vi "test_outfrq_fpga_1x_clc.vi"() -> ()   [LabVIEW 2013]
uses:
  <vilib>/Platform/TimedLoop/XDataNode/timing_clust.ctl
  <vilib>/Platform/TimedLoop/XDataNode/nitl_modes.ctl
  <vilib>/Platform/TimedLoop/XDataNode/wakeup.ctl
  <vilib>/rvi/Emulation/niFpgaSctlEmulationGetInTimedLoop.vi
  <vilib>/rvi/Emulation/niFpgaEmulationReportErrorSimple.vi
  <vilib>/rvi/Emulation/niFpgaGetClockAttributes.vi
  <vilib>/rvi/eio/common/nirviEmuTemplateMethod_errors.vi
  <vilib>/rvi/Emulation/niFpgaCriticalErrorInLSC.vi
  <vilib>/Platform/TimedLoop/XDataNode/XDataNode.xnode
  <vilib>/eio/EIONode/EIONode.xnode
  <vilib>/Platform/TimedLoop/XDataNode/XDNodeRunTimeDep.lvlib
panel:
  out "IO Module\\User Error":u8
  in  "use AO1":bool
  in  "User Command Commit":bool
  in  "User Command":u8
  out "User Command Idle":bool
  out "User Command Status":u8
  in  "User Data 0":u8
  in  "User Data 1":u8
  out "PLL Locked":bool
  out "Configured?":bool
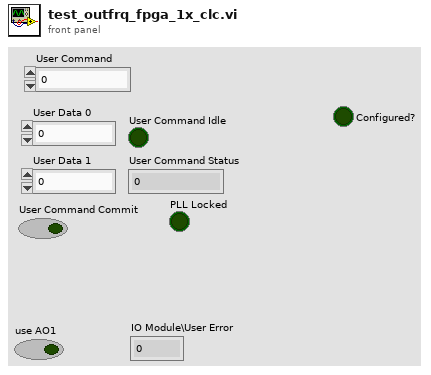
[diagram p1: front panel]
types:
  T1 = typedef "XDNodeRunTimeDep.lvlib/timing_clust.ctl" = cluster{"Expected End [f-1]":u64, "Actual End [f-1]":u64, "Finished Late? [f-1]":bool, "Expected End [i-1]":u64, "Actual End [i-1]":u64, "Finished Late? [i-1]":bool, "Expected Start [i]":u64, "Actual Start [i]":u64, "Expected Start [f]":u64, "Actual Start [f]":u64, "Source Name":string, "Structure Name":string, "Period":i64, "Deadline":i64, "Offset":i64, "Start":i64, "Priority":i32, "Timeout":i32, "Mode":T2, "Wakeup Reason":T3, "Error":errorcluster, "Source Type":string, "Secondary Source Type":string, "Global End Time":u64, "Global Start Time":u64, "Frame Duration":u64, "Iteration Duration":u64, "Assigned CPU":i32, "I/O Scan Engine Mode":u32}
  T2 = typedef "XDNodeRunTimeDep.lvlib/nitl_modes.ctl" = enum32{"No Change", "Process missed periods, maintain original phase", "Discard missed periods, maintain original phase", "Process missed periods, ignore original phase", "Discard missed periods, ignore original phase"}
  T3 = typedef "XDNodeRunTimeDep.lvlib/wakeup.ctl" = enum32{"Normal", "Aborted", "Asynchronous wakeup", "Timing source error", "Timed loop error", "Timeout"}
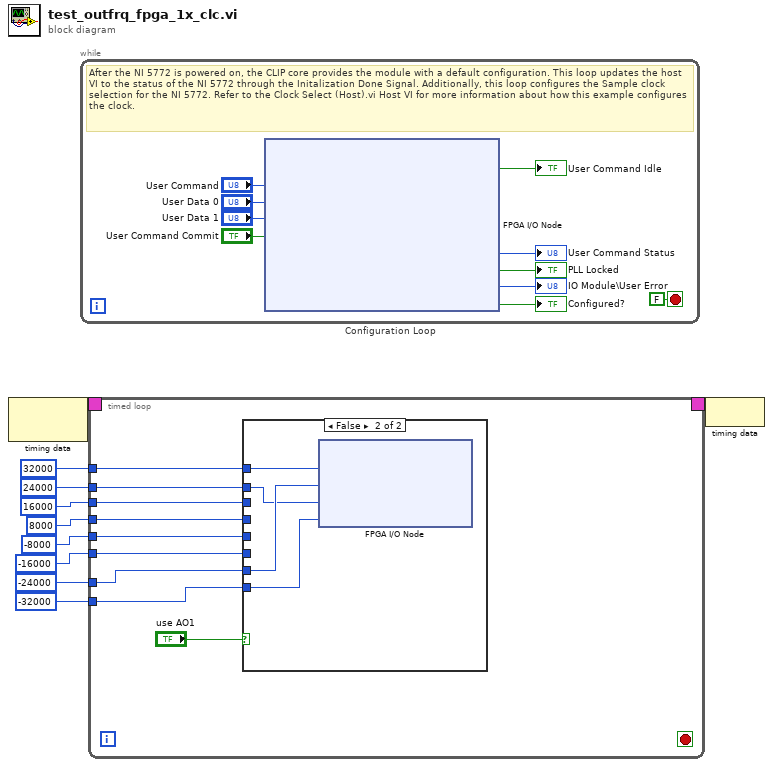
[diagram p0: block diagram]
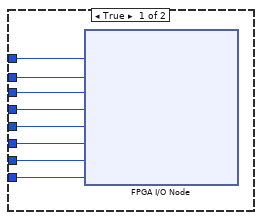
[diagram p2: hidden frame]
diagram:
  n1 = node-c288() -> (w10:T1)  [unwired: 1 in]
  n2 = while "Configuration Loop" {
    stop <- FALSE stop-if-true
    # "After the NI 5772 is powered on, the CLIP core provides the module with a default configuration. This loop updates the host VI to the status of the NI 5772 through the Initalization Done Signal. Additionally, this loop configures the Sample clock selection for the NI 5772. Refer to the Clock Select (Host).vi Host VI for more information about how this example configures the clock."
    n3 = xnode "FPGA I/O Node"("IO Module\\User Command"="User Command", "IO Module\\User Data 0"="User Data 0", "IO Module\\User Data 1"="User Data 1", "IO Module\\User Command Commit"="User Command Commit") -> ("IO Module\\User Command Idle"=→"User Command Idle":bool, "IO Module\\User Command Status"=→"User Command Status":u8, "IO Module\\PLL Locked"=→"PLL Locked":bool, "IO Module\\User Error"=→"IO Module\\User Error":u8, "IO Module\\Initialization Done"=→"Configured?":bool)  [unwired: 9 in, 9 out]
  }
  n4 = timed-loop {
    timing: w10 -> [_]
    timing-out: [_] -> w9
    tunnel: i16 32000 ("samples per period") -> [w29]
    tunnel: i16 24000 ("samples per period") -> [w28]
    tunnel: i16 16000 ("samples per period") -> [w27]
    tunnel: i16 8000 ("samples per period") -> [w26]
    tunnel: i16 -8000 ("samples per period") -> [w25]
    tunnel: i16 -16000 ("samples per period") -> [w24]
    tunnel: i16 -24000 ("samples per period") -> [w23]
    tunnel: i16 -32000 ("samples per period") -> [w22]
    stop <- _ stop-if-true
    n5 = case shown="False" "use AO1" {
      tunnel: w29 -> [w37 w41]
      tunnel: w28 -> [w36 w39]
      tunnel: w27 -> [w35 _]
      tunnel: w26 -> [w34 _]
      tunnel: w25 -> [w33 _]
      tunnel: w24 -> [w32 _]
      tunnel: w23 -> [w31 w40]
      tunnel: w22 -> [w30 w38]
      frame True {
        n6 = xnode "FPGA I/O Node"("IO Module\\AO 0 N-3"=w37, "IO Module\\AO 0 N-2"=w36, "IO Module\\AO 0 N-1"=w35, "IO Module\\AO 0 N"=w34, "IO Module\\AO 1 N-3"=w33, "IO Module\\AO 1 N-2"=w32, "IO Module\\AO 1 N-1"=w31, "IO Module\\AO 1 N"=w30) -> ()  [unwired: 8 in, 8 out]
      }
      frame False {
        n7 = xnode "FPGA I/O Node"("IO Module\\AO 0 N-3"=w41, "IO Module\\AO 0 N-2"=w40, "IO Module\\AO 0 N-1"=w39, "IO Module\\AO 0 N"=w38) -> ()  [unwired: 4 in, 4 out]
      }
    }
  }
  n8 = node-c288(w9) -> ()
